vi "save_ubin_tag.vi"(8 "error in":errorcluster, 10 "Name":string, 11 "refnum":refnum<file>) -> (0 "error out":errorcluster, 3 "refnum out":refnum<file>)   [LabVIEW 2012]
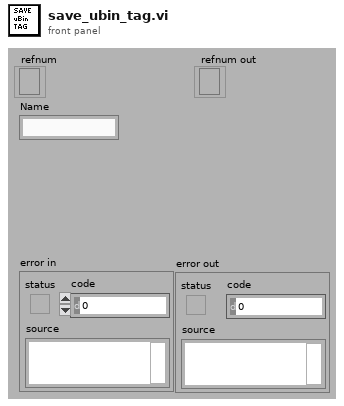
[diagram p1: front panel]
types:
  T1 = enum16{"big-endian, network order", "native, host order", "little-endian"}
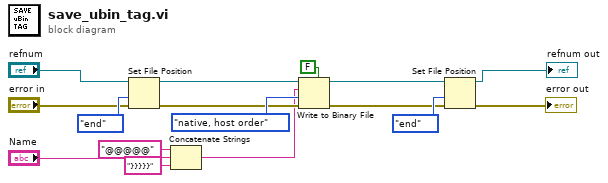
[diagram p0: block diagram]
diagram:
  n1 = Set File Position(refnum="refnum", from (0:start)=enum16{"start", "end", "current"}."end", error in="error in") -> (refnum out=w14:refnum<file>, error out=w9:errorcluster)  [unwired: 1 in]
  n2 = Concatenate Strings("@@@@@" ("string"), "Name", "}}}}}" ("string")) -> (w1:string)
  n3 = Write to Binary File(file (use dialog)=w14, data=w1, error in=w9, 5:FALSE ("prepend array or string size? (T)"), 9:T1."native, host order" ("byte order (0:big-endian, network order)")) -> (refnum out=w11:refnum<file>, error out=w8:errorcluster)  [unwired: 1 in, 1 out]
  n4 = Set File Position(refnum=w11, from (0:start)=enum16{"start", "end", "current"}."end", error in=w8) -> (refnum out=→"refnum out":refnum<file>, error out=→"error out":errorcluster)  [unwired: 1 in]
